vi "SistemaSisterna.vi"() -> ()   [LabVIEW 2010]
uses:
  <vilib>/Platform/TimedLoop/XDataNode/XDataNode.xnode
  <vilib>/Platform/TimedLoop/XDataNode/timing_clust.ctl
  <vilib>/Platform/TimedLoop/XDataNode/nitl_modes.ctl
  <vilib>/Platform/TimedLoop/XDataNode/wakeup.ctl
  <vilib>/Instr/_visa.llb/VISA Configure Serial Port (Instr).vi
  <vilib>/Platform/TimedLoop/XDataNode/XDNodeRunTimeDep.lvlib
panel:
  out "Tanque":dbl(slide) scale=0.0..18.0
  in  "Altura (cm)":u8(slide) scale=0.0..18.0
  in  "Period                :":i64=1000
  in  "Flow control    :":u16(ring) items=["None"=0, "XON/XOFF"=1, "RTS/CTS"=2, "DTR/DSR"=4]
  in  "Stop bits         :":u16(ring)=10 items=["1.0"=10, "1.5"=15, "2.0"=20]
  in  "Paridad            :":u16(ring) items=["None", "Odd", "Even", "Mark", "Space"]
  in  "Data bits          :":u16=8 min=5 max=8 step=1
  in  "VISA resource : name:":refnum<visa-resource-name>="COM1"
  in  "Baud rate         :":u32=9600
  in  "stop":bool
  out "Read buffer":string
  out "var t":i32
  # "Sisterna"
  # "Configuracion Serial"
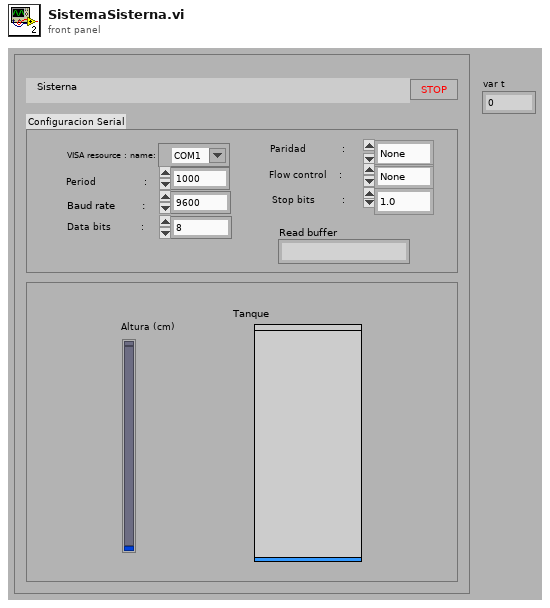
[diagram p1: front panel]
types:
  T1 = typedef "XDNodeRunTimeDep.lvlib/timing_clust.ctl" = cluster{"Expected End [f-1]":u64, "Actual End [f-1]":u64, "Finished Late? [f-1]":bool, "Expected End [i-1]":u64, "Actual End [i-1]":u64, "Finished Late? [i-1]":bool, "Expected Start [i]":u64, "Actual Start [i]":u64, "Expected Start [f]":u64, "Actual Start [f]":u64, "Source Name":string, "Structure Name":string, "Period":i64, "Deadline":i64, "Offset":i64, "Start":i64, "Priority":i32, "Timeout":i32, "Mode":T2, "Wakeup Reason":T3, "Error":errorcluster, "Source Type":string, "Secondary Source Type":string, "Global End Time":u64, "Global Start Time":u64, "Frame Duration":u64, "Iteration Duration":u64, "Assigned CPU":i32, "I/O Scan Engine Mode":u32}
  T2 = typedef "XDNodeRunTimeDep.lvlib/nitl_modes.ctl" = enum32{"No Change", "Process missed periods, maintain original phase", "Discard missed periods, maintain original phase", "Process missed periods, ignore original phase", "Discard missed periods, ignore original phase"}
  T3 = typedef "XDNodeRunTimeDep.lvlib/wakeup.ctl" = enum32{"Normal", "Aborted", "Asynchronous wakeup", "Timing source error", "Timed loop error", "Timeout"}
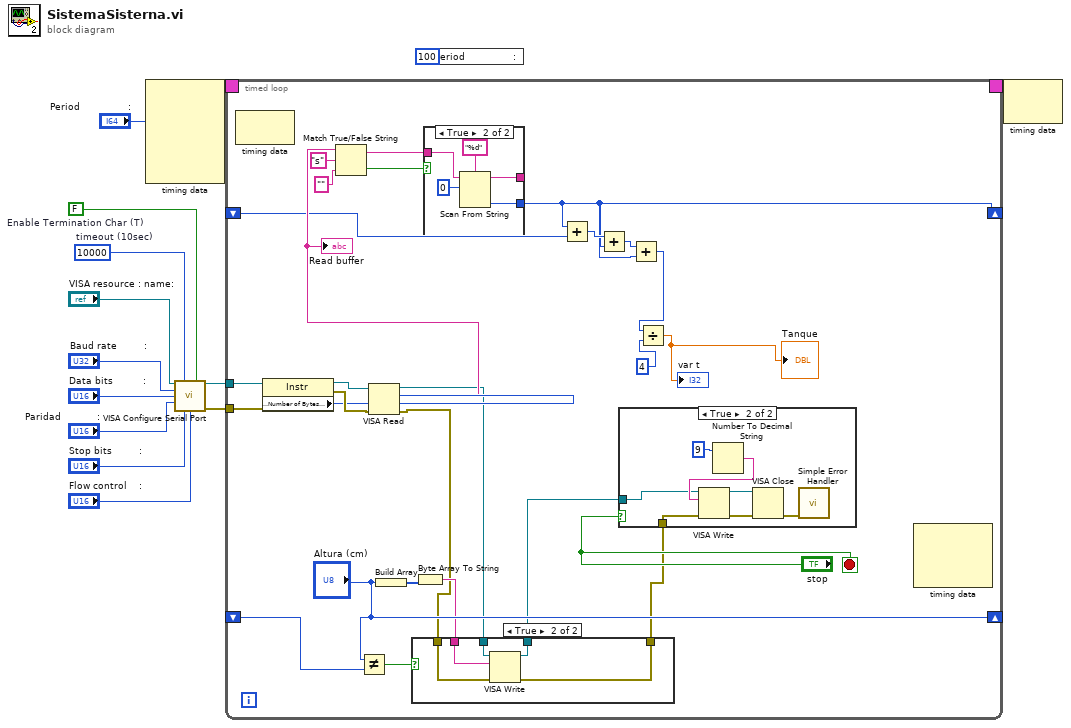
[diagram p0: block diagram]
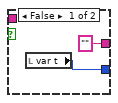
[diagram p3: hidden frame]
diagram:
  w8 = FALSE  # Enable Termination Char (T)
  w9 = u32 10000  # timeout (10sec)
  n1 = node-c288("Period                :") -> (w14:T1)  [unwired: 4 in]
  n2 = call-poly "VISA Configure Serial Port"("VISA resource name"="VISA resource : name:", "timeout (10sec)"=w9, "Enable Termination\nChar (T)"=w8, "baud rate (9600)"="Baud rate         :", "data bits (8)"="Data bits          :", "parity (0:none)"="Paridad            :", "stop bits (10: 1 bit)"="Stop bits         :", "flow control (0:none)"="Flow control    :") -> ("VISA resource name out"=w4:refnum<visa-resource-name>, "error out"=w3:errorcluster)  [unwired: 6 in]
  n3 = timed-loop {
    timing: w14 -> [_]
    timing-out: [_] -> w13
    tunnel: w4 -> [w32]
    tunnel: w3 -> [w31]
    shift-right: ["Altura (cm)"] -> _
    shift-left: _ -> [w27]
    shift-right: [w16] -> _
    shift-left: _ -> [w21]
    stop <- "stop" stop-if-true
    n4 = node-c288() -> ()  [unwired: 1 in, 1 out]
    n5 = property class="Instr"(reference=w32, error in=w31) -> (reference out=w33:refnum<visa-resource-name>, error out=w41:errorcluster, "Serial Settings:Number of Bytes at Serial Port"=w40:u32)
    n6 = Not Equal?(x="Altura (cm)", y=w27) -> (x != y?=w29:bool)
    n7 = VISA Read(VISA resource name=w33, byte count=w40, error in (no error)=w41) -> (VISA resource name out=w26:refnum<visa-resource-name>, read buffer=w38:string, error out=w24:errorcluster)  [unwired: 1 out]
    "Read buffer" <- w38
    n8 = Match True/False String(2:"" ("false string"), 3:"s" ("true string"), 4:w38) -> (0:w36:bool, 1:w35:string)
    n9 = Build Array("Altura (cm)") -> (w30:u8[])
    n10 = Byte Array To String(unsigned byte array=w30) -> (string=w25:string)
    n11 = case shown="True" w29 {
      tunnel: w26 -> [w43 w48]
      tunnel: w25 -> [_ w47]
      tunnel: w24 -> [w42 w46]
      tunnel: [w43 w45] -> w23
      tunnel: [w42 w44] -> w22
      frame False {
      }
      frame True {
        n12 = VISA Write(VISA resource name=w48, write buffer=w47, error in (no error)=w46) -> (VISA resource name out=w45:refnum<visa-resource-name>, error out=w44:errorcluster)  [unwired: 1 out]
      }
    }
    n13 = case shown="True" w36 {
      tunnel: w35 -> [_ w53]
      tunnel: ["" w52] -> _
      tunnel: [w50 w51] -> w16
      frame False {
        n14 = local read "var t"() -> (w50:i32)
      }
      frame True {
        n15 = Scan From String(format string="%d", input string=w53, initial scan location=u32 0) -> (remaining string=w52:string, output 1=w51:i32)  [unwired: 2 in, 2 out]
      }
    }
    n16 = Add(x=w16, y=w21) -> (x+y=w19:i32)
    n17 = Add(x=w19, y=w16) -> (x+y=w17:i32)
    n18 = case shown="True" "stop" {
      tunnel: w23 -> [_ w57]
      tunnel: w22 -> [_ w56]
      frame False {
      }
      frame True {
        n19 = Number To Decimal String(number=9) -> (decimal integer string=w58:string)  [unwired: 1 in]
        n20 = VISA Write(VISA resource name=w57, write buffer=w58, error in (no error)=w56) -> (VISA resource name out=w60:refnum<visa-resource-name>, error out=w59:errorcluster)  [unwired: 1 out]
        n21 = VISA Close(VISA resource name=w60, error in (no error)=w59) -> (error out=w62:errorcluster)
        n22 = call <vilib>:"Simple Error Handler.vi"("error in (no error)"=w62) -> ()  [unwired: 4 in, 5 out]
      }
    }
    n23 = Add(x=w17, y=w16) -> (x+y=w15:i32)
    n24 = Divide(x=w15, y=4) -> (x/y=→"var t" →"Tanque":dbl)
    n25 = node-c288() -> ()  [unwired: 3 in, 1 out]
  }
  n26 = local write "Period                :"(i64 100 ("Period")) -> ()
  n27 = node-c288(w13) -> ()  [unwired: 1 out]
